vi "Sequence Raffling.vi"(8 "error in (no error)":errorcluster, 10 "Number of Raffles":i32, 11 "GameLogic in":refnum<class "GameLogic.lvclass">) -> (0 "error out":errorcluster, 3 "GameLogic out":refnum<class "GameLogic.lvclass">)   [LabVIEW 2019, in "GameLogic.lvlib" / "GameLogic.lvclass"]
uses:
  GameLogic.lvclass
  GameLogic.lvclass/GameLogic.ctl
  <vilib>/numeric/Random Number (Range) U64.vi
  <vilib>/numeric/sub_Random U32.vi
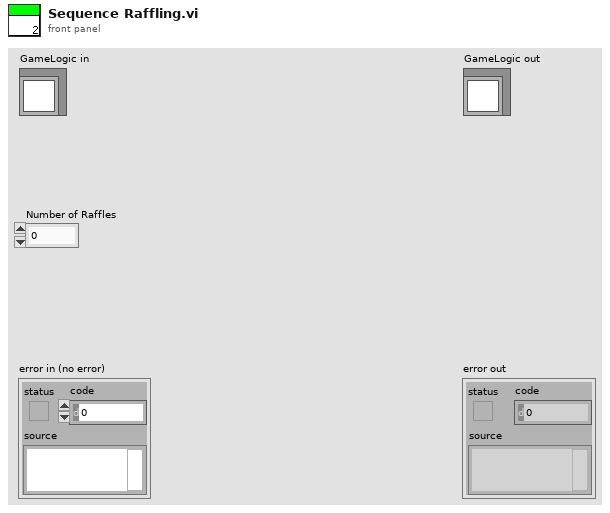
[diagram p1: front panel]
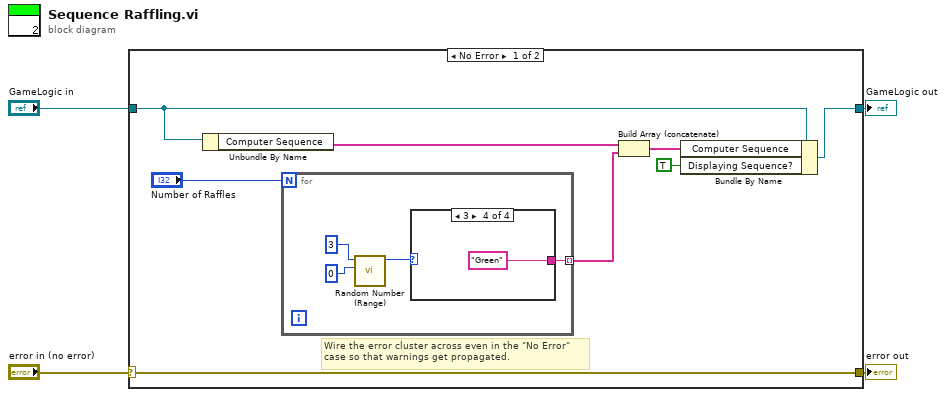
[diagram p0: block diagram]
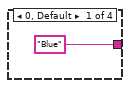
[diagram p2: hidden frame]
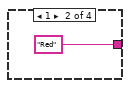
[diagram p3: hidden frame]
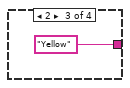
[diagram p4: hidden frame]
diagram:
  n1 = case shown="No Error" "error in (no error)" {
    selector: "error in (no error)" -> [w12 w22]
    tunnel: [w12 w22] -> w3
    tunnel: [w6 w21] -> w1
    tunnel: "GameLogic in" -> [w5 w21]
    frame No Error {
      # "Wire the error cluster across even in the \"No Error\"\ncase so that warnings get propagated."
      n2 = Unbundle By Name(w5) -> ("Computer Sequence"=w10:string[])
      n3 = for {
        N: "Number of Raffles" -> [_]
        tunnel: [w13] -> w9 mode=indexing
        n4 = call-poly <vilib>:"Random Number (Range).vi"("lower bound (0)"=u64 0, "upper bound (100)"=u64 3) -> ("number"=w14:u64)  [unwired: 9 in]
        n5 = case shown="3" w14 {
          tunnel: ["Blue" "Red" "Yellow" "Green"] -> w13
          frame 0, Default {
          }
          frame 1 {
          }
          frame 2 {
          }
          frame 3 {
          }
        }
      }
      n6 = Build Array (concatenate)(w10, w9) -> (w8:string[])
      n7 = Bundle By Name(cluster=w5, "Computer Sequence"=w8, "Displaying Sequence?"=TRUE) -> (w6:refnum<class "GameLogic.lvclass">)
    }
    frame Error {
    }
  }
  "error out" <- w3
  "GameLogic out" <- w1
